vi "VALUE_CHANGE4.vi"(8 "error in (no error)":errorcluster, 11 "Numeric":u16) -> (0 "error out":errorcluster, 3 "Boolean":bool)   [LabVIEW 2017]
uses:
  <userlib>/_OpenG.lib/comparison/comparison.llb/U16 Changed__ogtk.vi
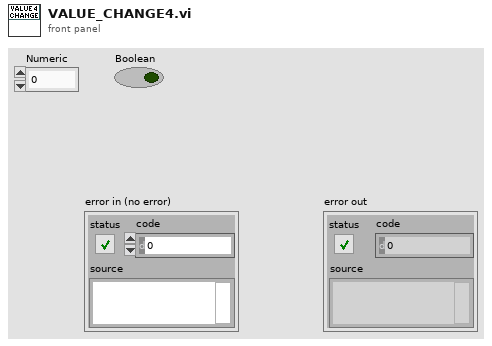
[diagram p1: front panel]
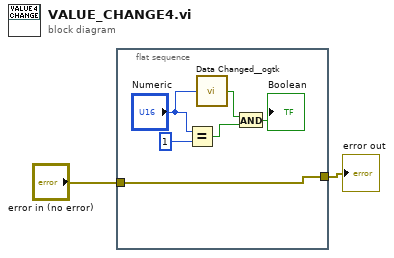
[diagram p0: block diagram]
diagram:
  n1 = flat-sequence {
    tunnel: [w4] -> w2
    tunnel: "error in (no error)" -> [w4]
    frame #0 {
      n2 = Equal?(x="Numeric", y=u16 1) -> (x = y?=w6:bool)
      n3 = call-poly <userlib>:"Data Changed__ogtk.vi"("U16"="Numeric") -> ("Changed"=w5:bool)
      n4 = And(x=w5, y=w6) -> (x .and. y?=→"Boolean":bool)
    }
  }
  "error out" <- w2
